vi "Set AO Channel Scale Offset (Public).vi"(8 "error in (no error)":errorcluster, 9 "ScaleOffset":dbl, 10 "AO":T1, 11 "DAQ":refnum<class "DAQ.lvclass">) -> (0 "error out":errorcluster, 3 "DAQ":refnum<class "DAQ.lvclass">)   [LabVIEW 2017, in "DAQ.lvclass"]
doc: "Developed by Kevin Thompson\nkevin@thompsonengineering.net\n\nCopyright 2018-2020\nThompson Engineering, LLC"
uses:
  DAQ.lvclass
  DataTypes/TD AO IOName--enum.ctl
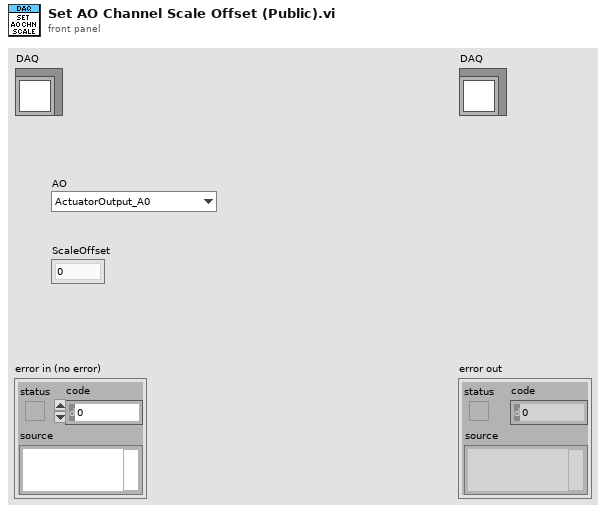
[diagram p1: front panel]
types:
  T1 = typedef "DAQ.lvclass/TD AO IOName--enum.ctl" = enum16{"ActuatorOutput_A0"}
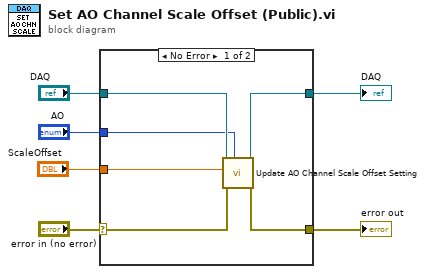
[diagram p0: block diagram]
diagram:
  n1 = case shown="No Error" "error in (no error)" {
    selector: "error in (no error)" -> [w12 w14]
    tunnel: [w11 w14] -> w5
    tunnel: [w9 w13] -> w3
    tunnel: "DAQ" -> [w10 w13]
    tunnel: "AO" -> [w8 _]
    tunnel: "ScaleOffset" -> [w7 _]
    frame No Error {
      n2 = call "Update AO Channel Scale Offset Setting.vi"("IOName (enum)"=w8, "error in (no error)"=w12, "ScaleOffset"=w7, "DAQ"=w10) -> ("error out"=w11:errorcluster, "DAQ"=w9:refnum<class "DAQ.lvclass">)  [unwired: 5 in, 1 out]
    }
    frame Error {
    }
  }
  "error out" <- w5
  "DAQ" <- w3
